vi "Lorentzian complex bg test Jacobian.vi"(3 "output control":T1, 4 "data":variant, 5 "X":dbl[](array[numeric]) format="%#_10g", 6 "a":dbl[](array[numeric])) -> (0 "error out":errorcluster, 1 "f'(X,a)":dbl[][](array[numeric]), 2 "f(X,a)":dbl[](array[numeric]))   [LabVIEW 2016]
doc: "Sum of three Gaussians, plus DC offset."
uses:
  <vilib>/gmath/NumericalOptimization/LM_output select.ctl
  <vilib>/gmath/NI_Gmath.lvlib
panel:
  out "Waveform Graph":dbl[][](graph)
  # "F0\nG\nA\nP\nX\nY"
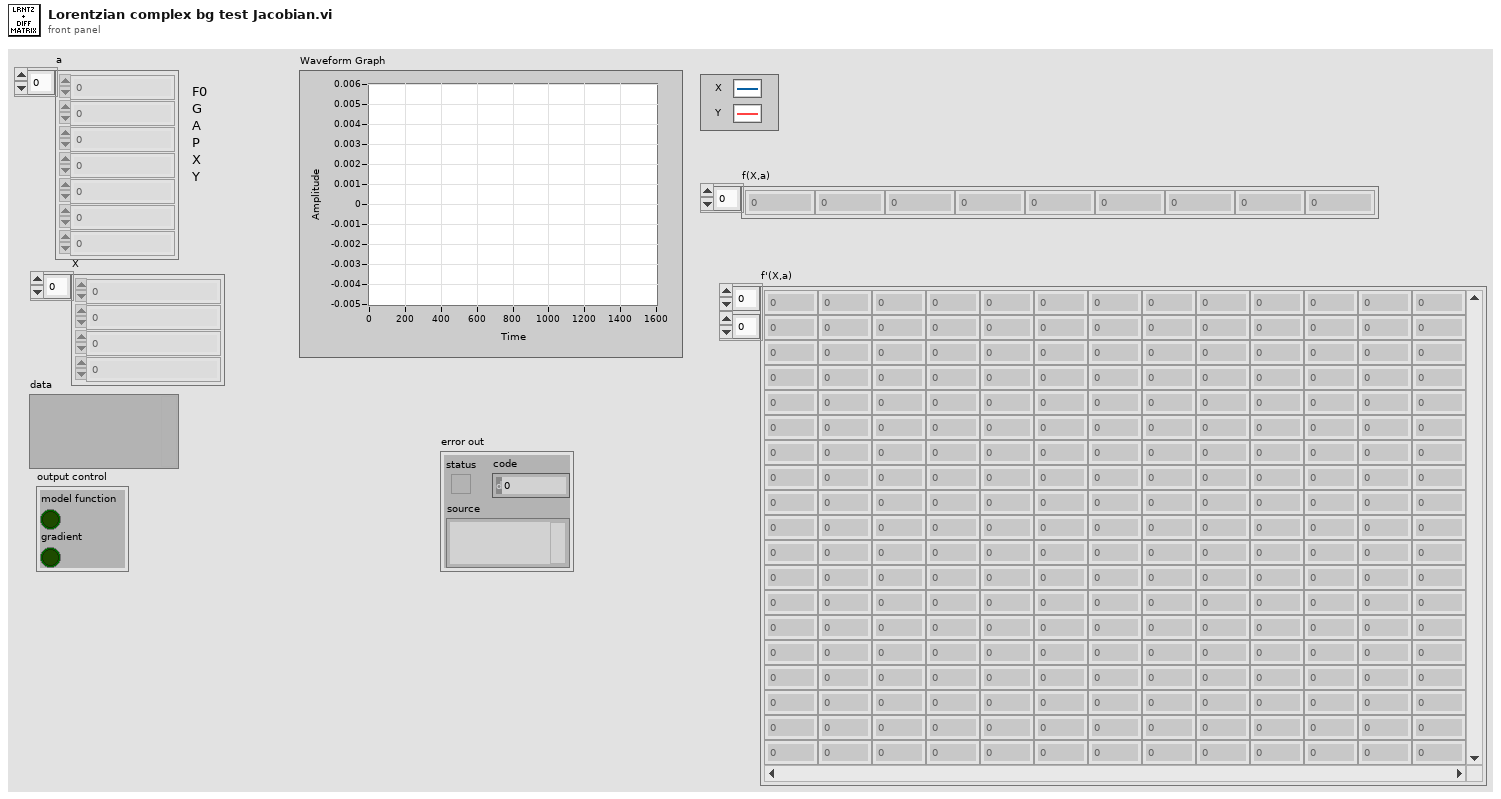
[diagram p1: front panel]
types:
  T1 = typedef "NI_Gmath.lvlib/LM_output select.ctl" = cluster{"model function":bool, "gradient":bool}
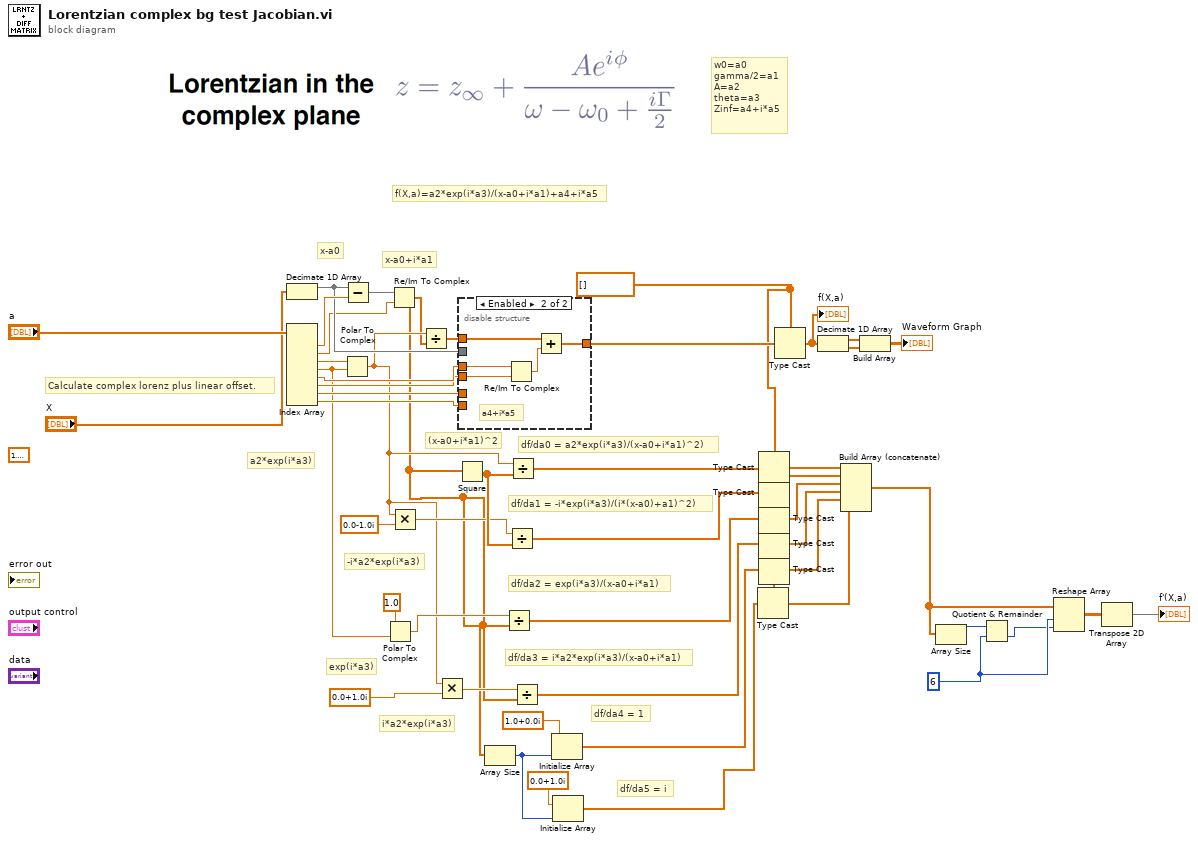
[diagram p0: block diagram]
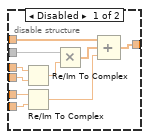
[diagram p2: hidden frame]
diagram:
  w18 = 6 ("dimension size")
  (unwired) 1.5707963267948966
  w6 = dbl[] []
  # "i*a2*exp(i*a3)"
  # "exp(i*a3)"
  # "w0=a0\ngamma/2=a1\nA=a2\ntheta=a3\nZinf=a4+i*a5"
  # "-i*a2*exp(i*a3)"
  # "(x-a0+i*a1)^2"
  # "x-a0+i*a1"
  # "x-a0"
  # "a2*exp(i*a3)"
  # "df/da5 = i"
  # "df/da4 = 1"
  # "df/da3 = i*a2*exp(i*a3)/(x-a0+i*a1)"
  # "df/da2 = exp(i*a3)/(x-a0+i*a1)"
  # "df/da1 = -i*exp(i*a3)/(i*(x-a0)+a1)^2)"
  # "df/da0 = a2*exp(i*a3)/(x-a0+i*a1)^2)"
  # "f(X,a)=a2*exp(i*a3)/(x-a0+i*a1)+a4+i*a5"
  # "Calculate complex lorenz plus linear offset."
  n1 = Decimate 1D Array("X") -> (w40:dbl[])  [unwired: 1 out]
  n2 = Index Array(array="a") -> (element #1=w48:dbl, element #2=w29:dbl, element #3=w47:dbl, element #4=w32:dbl, element #5=w46:dbl, element #6=w45:dbl, element #7=w43:dbl, element #8=w42:dbl)  [unwired: 8 in]
  n3 = Polar To Complex(1:w32, 2:w47) -> (0:w25:cdb)
  n4 = Subtract(x=w40, y=w48) -> (x-y=w30:dbl[])
  n5 = Polar To Complex(1:w32, 2:1.0 ("r")) -> (0:w27:cdb)
  n6 = Re/Im To Complex(1:w29, 2:w30) -> (0:w23:cdb[])
  n7 = Multiply(x=w25, y=cdb 0.0-1.0i) -> (x*y=w28:cdb)
  n8 = Divide(x=w25, y=w23) -> (x/y=w41:cdb[])
  n9 = Multiply(x=w25, y=cdb 0.0+1.0i) -> (x*y=w24:cdb)
  n10 = Square(x=w23) -> (x^2=w33:cdb[])
  n11 = disable-structure shown="Enabled" {
    disable-tunnel: w46 -> [w59 w64]
    disable-tunnel: w45 -> [w58 w63]
    disable-tunnel: w43 -> [w55 _]
    disable-tunnel: w42 -> [w54 _]
    disable-tunnel: w41 -> [w52 w62]
    disable-tunnel: [w51 w61] -> w39
    disable-tunnel: w40 -> [w50 _]
    frame Disabled {
      n12 = Re/Im To Complex(1:w58, 2:w59) -> (0:w57:cdb)
      n13 = Re/Im To Complex(1:w54, 2:w55) -> (0:w53:cdb)
      n14 = Multiply(x=w50, y=w57) -> (x*y=w56:cdb[])
      n15 = Compound Arithmetic op=ADD(w52, w56, w53) -> (w51:cdb[])
    }
    frame Enabled {
      # "a4+i*a5"
      n16 = Re/Im To Complex(1:w63, 2:w64) -> (0:w60:cdb)
      n17 = Add(x=w62, y=w60) -> (x+y=w61:cdb[])
    }
  }
  n18 = Array Size(array=w23) -> (size(s)=w20:i32)
  n19 = Divide(x=w27, y=w23) -> (x/y=w12:cdb[])
  n20 = Divide(x=w28, y=w33) -> (x/y=w14:cdb[])
  n21 = Divide(x=w25, y=w33) -> (x/y=w16:cdb[])
  n22 = Divide(x=w24, y=w23) -> (x/y=w9:cdb[])
  n23 = Initialize Array(cdb 1.0+0.0i ("y"), w20) -> (w8:cdb[])
  n24 = Initialize Array(cdb 0.0+1.0i ("y"), w20) -> (w5:cdb[])
  n25 = Type Cast(type=w6, x=w5) -> (*(type *) &x=w4:dbl[])
  n26 = Type Cast(type=w6, x=w16) -> (*(type *) &x=w15:dbl[])
  n27 = Type Cast(type=w6, x=w14) -> (*(type *) &x=w13:dbl[])
  n28 = Type Cast(type=w6, x=w12) -> (*(type *) &x=w11:dbl[])
  n29 = Type Cast(type=w6, x=w9) -> (*(type *) &x=w10:dbl[])
  n30 = Type Cast(type=w6, x=w8) -> (*(type *) &x=w7:dbl[])
  n31 = Type Cast(type=w6, x=w39) -> (*(type *) &x=w38:dbl[])
  "f(X,a)" <- w38
  n32 = Decimate 1D Array(w38) -> (w37:dbl[], w36:dbl[])
  n33 = Build Array (concatenate)(w15, w13, w11, w10, w7, w4) -> (w3:dbl[])
  n34 = Build Array(w37, w36) -> (→"Waveform Graph":dbl[][])
  n35 = Array Size(array=w3) -> (size(s)=w19:i32)
  n36 = Quotient & Remainder(x=w19, y=w18) -> (floor(x/y)=w17:i32)  [unwired: 1 out]
  n37 = Reshape Array(w3, w18, w17) -> (w2:dbl[][])
  n38 = Transpose 2D Array(2D array=w2) -> (transposed array=→"f'(X,a)":dbl[][])
